vi "set_in_library.vi"(2 "Cluster":T4, 3 "camera cluster":T3, 4 "Tracker Handle":i32, 5 "Array":dbl[][](array[numeric])) -> (0 "No Error":bool, 1 "Directory Exists?":bool)   [LabVIEW 2015]
uses:
  <vilib>/vision/Avi1.llb/AviRefnum.ctl
  <vilib>/userdefined/High Color/IMAQdx.ctl
  MWT.dll
panel:
  out "return type 9":i32
  out "return type 8":i32
  out "return type 7":i32
  out "return type 6":i32
  out "return type 5":i32
  out "return type 4":i32
  out "return type 3":i32
  out "return type 2":i32
  out "return type":i32
  in  "ObjectFrames of Persistence":i32=5
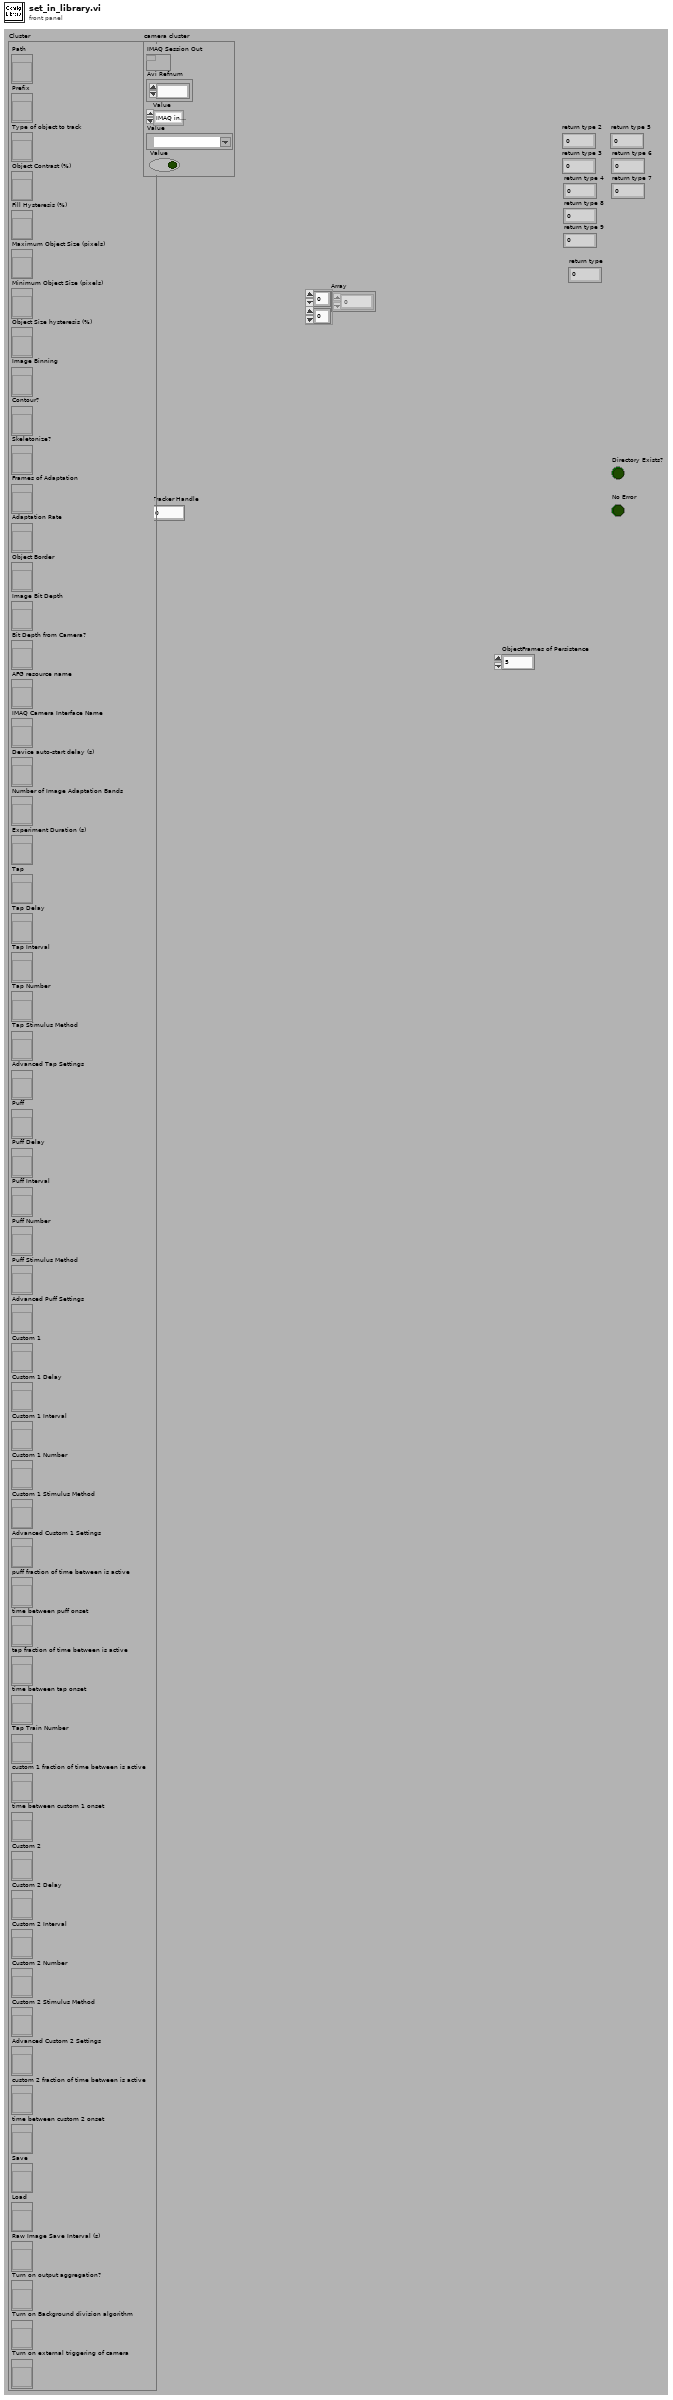
[diagram p1: front panel]
types:
  T1 = typedef "AviRefnum.ctl" = refnum<k1>
  T2 = typedef "IMAQdx.ctl" = refnum<k21>
  T3 = cluster{"IMAQ Session Out":refnum<k11>, "Avi Refnum":T1, "Value":enum32{"IMAQ interface", "IMAQdx interface", "AVI file"}, "Value":T2, "Value":bool}
  T4 = cluster{"Path":refnum<vi>, "Prefix":refnum<vi>, "Type of object to track":refnum<vi>, "Object Contrast (%)":refnum<vi>, "Fill Hysteresis (%)":refnum<vi>, "Maximum Object Size (pixels)":refnum<vi>, "Minimum Object Size (pixels)":refnum<vi>, "Object Size hysteresis (%)":refnum<vi>, "Image Binning":refnum<vi>, "Contour?":refnum<vi>, "Skeletonize?":refnum<vi>, "Frames of Adaptation":refnum<vi>, "Adaptation Rate":refnum<vi>, "Object Border":refnum<vi>, "Image Bit Depth":refnum<vi>, "Bit Depth from Camera?":refnum<vi>, "AFG resource name":refnum<vi>, "IMAQ Camera Interface Name":refnum<vi>, "Device auto-start delay (s)":refnum<vi>, "Number of Image Adaptation Bands":refnum<vi>, "Experiment Duration (s)":refnum<vi>, "Tap":refnum<vi>, "Tap Delay":refnum<vi>, "Tap Interval":refnum<vi>, "Tap Number":refnum<vi>, "Tap Stimulus Method":refnum<vi>, "Advanced Tap Settings":refnum<vi>, "Puff":refnum<vi>, "Puff Delay":refnum<vi>, "Puff Interval":refnum<vi>, "Puff Number":refnum<vi>, "Puff Stimulus Method":refnum<vi>, "Advanced Puff Settings":refnum<vi>, "Custom 1":refnum<vi>, "Custom 1 Delay":refnum<vi>, "Custom 1 Interval":refnum<vi>, "Custom 1 Number":refnum<vi>, "Custom 1 Stimulus Method":refnum<vi>, "Advanced Custom 1 Settings":refnum<vi>, "puff fraction of time between is active":refnum<vi>, "time between puff onset":refnum<vi>, "tap fraction of time between is active":refnum<vi>, "time between tap onset":refnum<vi>, "Tap Train Number":refnum<vi>, "custom 1 fraction of time between is active":refnum<vi>, "time between custom 1 onset":refnum<vi>, "Custom 2":refnum<vi>, "Custom 2 Delay":refnum<vi>, "Custom 2 Interval":refnum<vi>, "Custom 2 Number":refnum<vi>, "Custom 2 Stimulus Method":refnum<vi>, "Advanced Custom 2 Settings":refnum<vi>, "custom 2 fraction of time between is active":refnum<vi>, "time between custom 2 onset":refnum<vi>, "Save":refnum<vi>, "Load":refnum<vi>, "Raw Image Save Interval (s)":refnum<vi>, "Turn on output aggregation?":refnum<vi>, "Turn on Background division algorithm":refnum<vi>, "Turn on external triggering of camera":refnum<vi>}
  T5 = cluster{"Value":path, "Value":string, "Value":bool, "Value":dbl, "Value":dbl, "Value":i32, "Value":i32, "Value":dbl, "Value":u16, "Value":bool, "Value":bool, "Value":i32, "Value":i32, "Value":i32, "Value":u32, "Value":i32, "Value":bool}
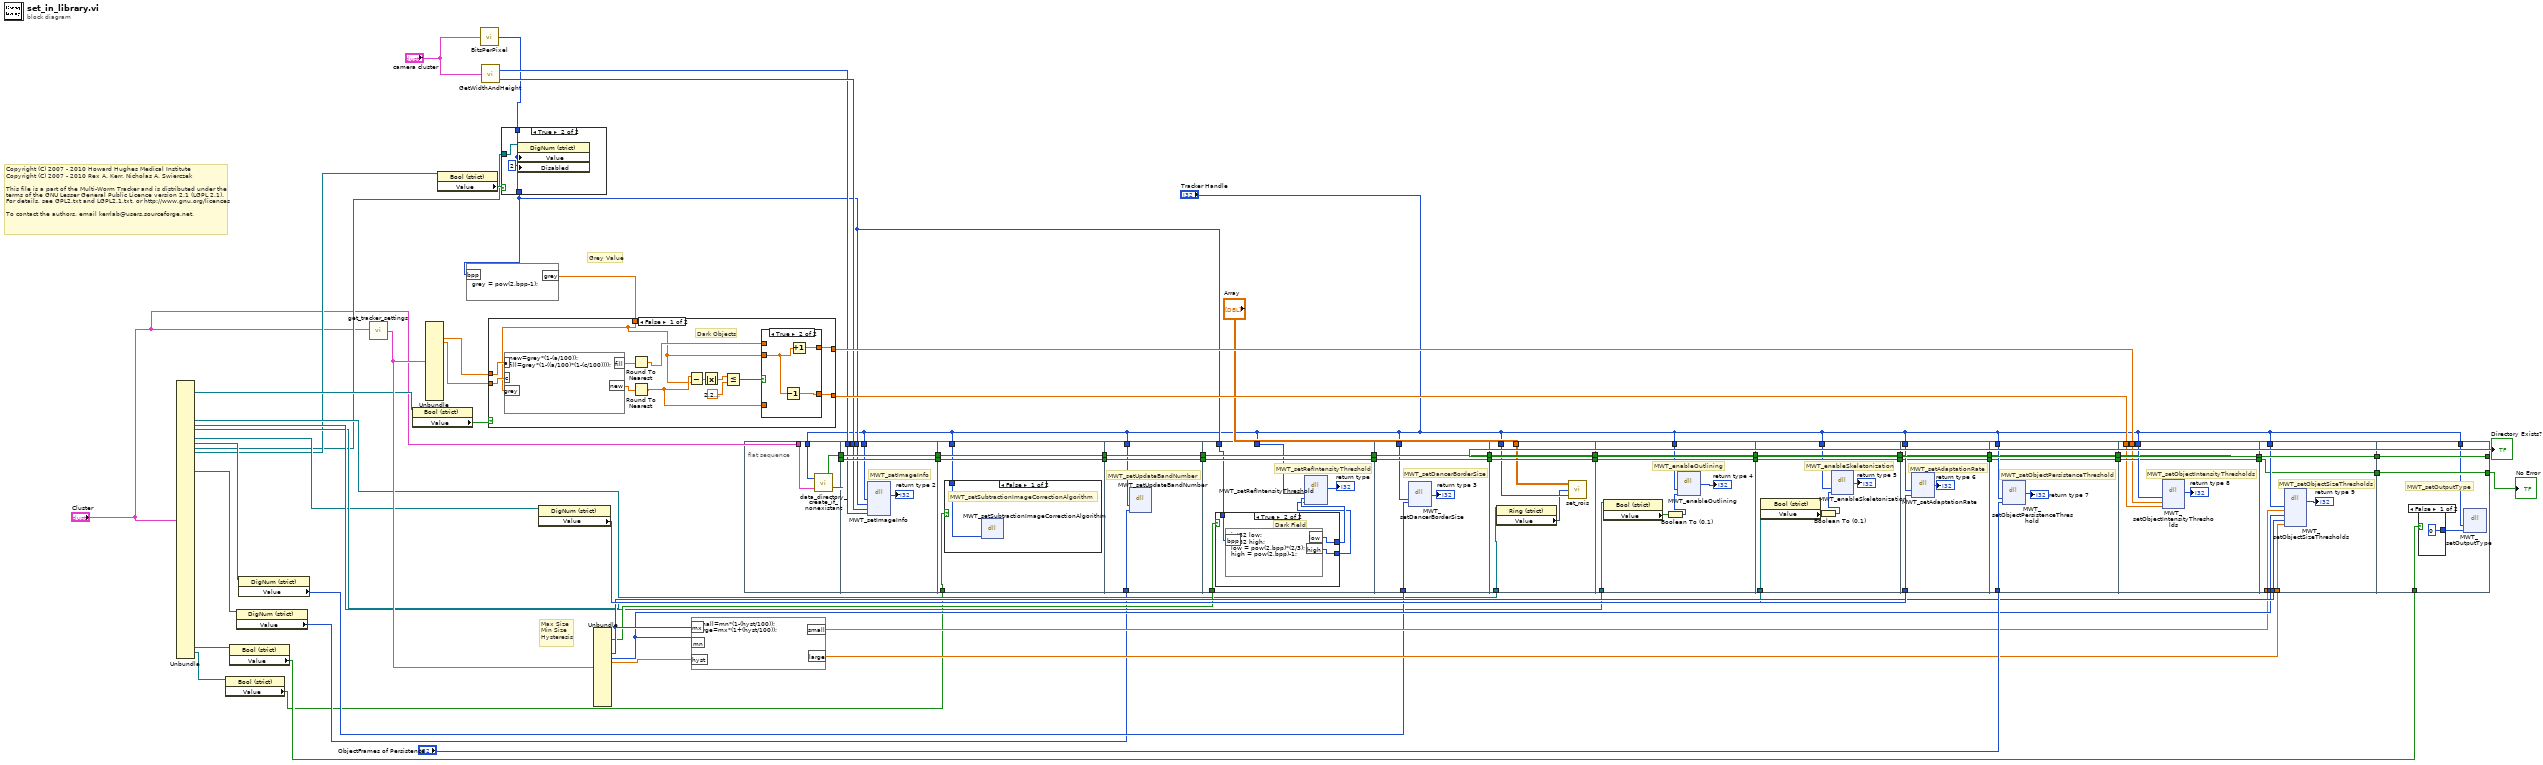
[diagram p0: block diagram]
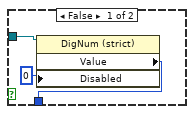
[diagram p2: hidden frame]
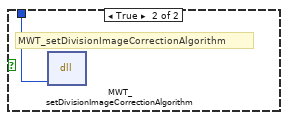
[diagram p3: hidden frame]
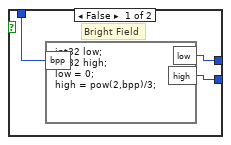
[diagram p4: hidden frame]
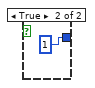
[diagram p5: hidden frame]
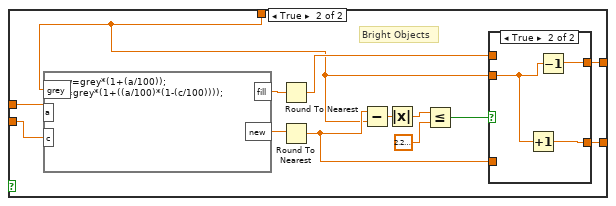
[diagram p7: hidden frame]
diagram:
  # "Copyright (C) 2007 - 2010 Howard Hughes Medical Institute\nCopyright (C) 2007 - 2010 Rex A. Kerr, Nicholas A. Swierczek\n \nThis file is a part of the Multi-Worm Tracker and is distributed under the\nterms of the GNU Lesser General Public Licence version 2.1 (LGPL 2.1).\nFor details, see GPL2.txt and LGPL2.1.txt, or http://www.gnu.org/licences\n \nTo contact the authors, email kerrlab@users.sourceforge.net."
  # "Max Size\nMin Size\nHysteresis"
  # "Grey Value"
  n1 = Unbundle("Cluster") -> ("Type of object to track"=w25:refnum<vi>, "Image Binning"=w24:refnum<vi>, "Contour?"=w23:refnum<vi>, "Skeletonize?"=w22:refnum<vi>, "Adaptation Rate"=w21:refnum<vi>, "Object Border"=w20:refnum<vi>, "Image Bit Depth"=w18:refnum<vi>, "Bit Depth from Camera?"=w19:refnum<vi>, "Number of Image Adaptation Bands"=w15:refnum<vi>, "Turn on output aggregation?"=w11:refnum<vi>, "Turn on Background division algorithm"=w5:refnum<vi>)  [unwired: 49 out]
  n2 = property class="Bool (strict)"(reference=w5) -> ("Value"=w4:bool)  [unwired: 1 in, 2 out]
  n3 = property class="Bool (strict)"(reference=w11) -> ("Value"=w10:bool)  [unwired: 1 in, 2 out]
  n4 = property class="DigNum (strict)"(reference=w15) -> ("Value"=w14:i32)  [unwired: 1 in, 2 out]
  n5 = property class="DigNum (strict)"(reference=w20) -> ("Value"=w31:i32)  [unwired: 1 in, 2 out]
  n6 = call "get_tracker_settings.vi"("Cluster"="Cluster") -> ("settings value cluster"=w66:T5)
  n7 = property class="Bool (strict)"(reference=w25) -> ("Value"=w67:bool)  [unwired: 1 in, 2 out]
  n8 = Unbundle(w66) -> ("Value"=w37:dbl, "Value"=w65:dbl)  [unwired: 15 out]
  n9 = property class="Bool (strict)"(reference=w19) -> ("Value"=w42:bool)  [unwired: 1 in, 2 out]
  n10 = call "BitsPerPixel.vi"("camera cluster"="camera cluster") -> ("BitsPerPixel"=w28:u32)
  n11 = call "GetWidthAndHeight.vi"("camera cluster"="camera cluster") -> ("Width"=w29:u32, "Height"=w30:u32)
  n12 = case shown="True" w42 {
    tunnel: [w69 w72] -> w27
    tunnel: w28 -> [_ w72]
    tunnel: w18 -> [w70 w73]
    frame False {
      n13 = property class="DigNum (strict)"(reference=w70, "Disabled"=u8 0) -> ("Value"=w69:u32)  [unwired: 1 in, 2 out]
    }
    frame True {
      n14 = property class="DigNum (strict)"(reference=w73, "Value"=w72, "Disabled"=u8 2) -> ()  [unwired: 1 in, 2 out]
    }
  }
  n15 = formula code="grey = pow(2,bpp-1);"("bpp"=w27) -> ("grey"=w43:dbl)
  n16 = case shown="False" w67 {
    tunnel: w43 -> [w74 w92]
    tunnel: w37 -> [w86 w104]
    tunnel: w65 -> [w85 w103]
    tunnel: [w77 w100] -> w64
    tunnel: [w78 w98] -> w63
    frame False {
      # "Dark Objects"
      n17 = formula code="new=grey*(1-(a/100));\nfill=grey*(1-((a/100)*(1-(c/100))));"("a"=w86, "c"=w85, "grey"=w74) -> ("new"=w84:dbl, "fill"=w83:dbl)
      n18 = Round To Nearest(number=w83) -> (nearest integer value=w76:dbl)
      n19 = Round To Nearest(number=w84) -> (nearest integer value=w75:dbl)
      n20 = Subtract(x=w75, y=w74) -> (x-y=w82:dbl)
      n21 = Absolute Value(x=w82) -> (abs(x)=w80:dbl)
      n22 = Less Or Equal?(x=w80, y=2.220446049250313e-16) -> (x <= y?=w81:bool)
      n23 = case shown="True" w81 {
        tunnel: [w88 w90] -> w77
        tunnel: w76 -> [w88 _]
        tunnel: [w87 w91] -> w78
        tunnel: w75 -> [w87 _]
        tunnel: w74 -> [_ w89]
        frame False {
        }
        frame True {
          n24 = Decrement(x=w89) -> (x-1=w91:dbl)
          n25 = Increment(x=w89) -> (x+1=w90:dbl)
        }
      }
    }
    frame True {
      # "Bright Objects"
      n26 = formula code="new=grey*(1+(a/100));\nfill=grey*(1+((a/100)*(1-(c/100))));"("a"=w104, "c"=w103, "grey"=w92) -> ("new"=w102:dbl, "fill"=w101:dbl)
      n27 = Round To Nearest(number=w101) -> (nearest integer value=w99:dbl)
      n28 = Round To Nearest(number=w102) -> (nearest integer value=w96:dbl)
      n29 = Subtract(x=w96, y=w92) -> (x-y=w97:dbl)
      n30 = Absolute Value(x=w97) -> (abs(x)=w94:dbl)
      n31 = Less Or Equal?(x=w94, y=2.220446049250313e-16) -> (x <= y?=w95:bool)
      n32 = case shown="True" w95 {
        tunnel: [w106 w108] -> w100
        tunnel: w99 -> [w106 _]
        tunnel: [w105 w109] -> w98
        tunnel: w96 -> [w105 _]
        tunnel: w92 -> [_ w107]
        frame False {
        }
        frame True {
          n33 = Increment(x=w107) -> (x+1=w109:dbl)
          n34 = Decrement(x=w107) -> (x-1=w108:dbl)
        }
      }
    }
  }
  n35 = property class="DigNum (strict)"(reference=w21) -> ("Value"=w62:i32)  [unwired: 1 in, 2 out]
  n36 = Unbundle(w66) -> ("Value"=w26:bool, "Value"=w36:i32, "Value"=w35:i32, "Value"=w34:dbl)  [unwired: 13 out]
  n37 = formula code="small=mn*(1-(hyst/100));\nlarge=mx*(1+(hyst/100));"("mx"=w36, "mn"=w35, "hyst"=w34) -> ("small"=w33:dbl, "large"=w32:dbl)
  n38 = flat-sequence {
    tunnel: [w113] -> w45
    tunnel: [w112] -> w44
    tunnel: "Tracker Handle" -> [w111]
    tunnel: "Cluster" -> [w110]
    tunnel: w45 -> [w120]
    tunnel: [w120] -> w9
    tunnel: w44 -> [w119]
    tunnel: [w119] -> w7
    tunnel: "Tracker Handle" -> [w118]
    tunnel: w27 -> [w117]
    tunnel: w29 -> [w116]
    tunnel: w30 -> [w115]
    tunnel: w9 -> [w124]
    tunnel: [w124] -> w8
    tunnel: w7 -> [w123]
    tunnel: [w123] -> w6
    tunnel: w4 -> [w122]
    tunnel: "Tracker Handle" -> [w121]
    tunnel: w8 -> [w130]
    tunnel: [w130] -> w17
    tunnel: w6 -> [w129]
    tunnel: [w129] -> w16
    tunnel: "Tracker Handle" -> [w128]
    tunnel: w14 -> [w127]
    tunnel: w17 -> [w138]
    tunnel: [w138] -> w49
    tunnel: w16 -> [w137]
    tunnel: [w137] -> w47
    tunnel: "Tracker Handle" -> [w136]
    tunnel: w27 -> [w133]
    tunnel: w26 -> [w134]
    tunnel: w49 -> [w149]
    tunnel: [w149] -> w48
    tunnel: w47 -> [w148]
    tunnel: [w148] -> w46
    tunnel: "Tracker Handle" -> [w147]
    tunnel: w31 -> [w146]
    tunnel: w48 -> [w155]
    tunnel: [w155] -> w41
    tunnel: w46 -> [w154]
    tunnel: [w154] -> w39
    tunnel: "Array" -> [w153]
    tunnel: "Tracker Handle" -> [w152]
    tunnel: w24 -> [w151]
    tunnel: w41 -> [w162]
    tunnel: [w162] -> w40
    tunnel: w39 -> [w161]
    tunnel: [w161] -> w38
    tunnel: "Tracker Handle" -> [w158]
    tunnel: w23 -> [w157]
    tunnel: [w169] -> w57
    tunnel: w40 -> [w169]
    tunnel: w38 -> [w168]
    tunnel: [w168] -> w56
    tunnel: "Tracker Handle" -> [w167]
    tunnel: w22 -> [w166]
    tunnel: w62 -> [w174]
    tunnel: "Tracker Handle" -> [w173]
    tunnel: [w172] -> w58
    tunnel: w57 -> [w172]
    tunnel: w56 -> [w171]
    tunnel: [w171] -> w55
    tunnel: "ObjectFrames of Persistence" -> [w179]
    tunnel: "Tracker Handle" -> [w178]
    tunnel: [w177] -> w59
    tunnel: w58 -> [w177]
    tunnel: w55 -> [w176]
    tunnel: [w176] -> w54
    tunnel: w64 -> [w181]
    tunnel: w63 -> [w182]
    tunnel: "Tracker Handle" -> [w185]
    tunnel: [w184] -> w60
    tunnel: w59 -> [w184]
    tunnel: w54 -> [w183]
    tunnel: [w183] -> w53
    tunnel: w33 -> [w193]
    tunnel: w35 -> [w192]
    tunnel: w36 -> [w191]
    tunnel: w32 -> [w190]
    tunnel: "Tracker Handle" -> [w189]
    tunnel: w60 -> [w188]
    tunnel: w53 -> [w187]
    tunnel: [w188] -> w13
    tunnel: [w187] -> w12
    tunnel: [w197] -> w51
    tunnel: [w198] -> w52
    tunnel: w13 -> [w198]
    tunnel: w12 -> [w197]
    tunnel: "Tracker Handle" -> [w195]
    tunnel: w10 -> [w194]
    frame #0 {
      n39 = call "data_directory_create_if_nonexistant.vi"("Cluster"=w110, "Tracker Handle"=w111) -> ("Error"=w112:bool, "Directory Exists?"=w113:bool)
    }
    frame #1 {
      # "MWT_setImageInfo"
      n40 = dll-call lib="C:/Users/ramasamyl/Desktop/MWT/MWT.dll" fn="MWT_setImageInfo"("handle"=w118, "bits"=w117, "width"=w115, "height"=w116) -> ("return type"=→"return type 2":i32)  [unwired: 7 in, 2 out]
    }
    frame #2 {
      n41 = case shown="False" w122 {
        tunnel: w121 -> [w125 w126]
        frame False {
          # "MWT_setSubtractionImageCorrectionAlgorithm"
          n42 = dll-call lib="C:/Users/ramasamyl/Desktop/MWT/MWT.dll" fn="MWT_setSubtractionImageCorrectionAlgorithm"("handle"=w125) -> ()  [unwired: 5 in, 2 out]
        }
        frame True {
          # "MWT_setDivisionImageCorrectionAlgorithm"
          n43 = dll-call lib="C:/Users/ramasamyl/Desktop/MWT/MWT.dll" fn="MWT_setDivisionImageCorrectionAlgorithm"("handle"=w126) -> ()  [unwired: 5 in, 2 out]
        }
      }
    }
    frame #3 {
      # "MWT_setUpdateBandNumber"
      n44 = dll-call lib="C:/Users/ramasamyl/Desktop/MWT/MWT.dll" fn="MWT_setUpdateBandNumber"("handle"=w128, "num_bands"=w127) -> ()  [unwired: 6 in, 2 out]
    }
    frame #4 {
      # "MWT_setRefIntensityThreshold"
      n45 = case shown="True" w134 {
        tunnel: [w141 w144] -> w132
        tunnel: [w140 w143] -> w131
        tunnel: w133 -> [w139 w142]
        frame False {
          # "Bright Field"
          n46 = formula code="int32 low;\nint32 high;\nlow = 0;\nhigh = pow(2,bpp)/3;"("bpp"=w139) -> ("low"=w141:i32, "high"=w140:i32)
        }
        frame True {
          # "Dark Field"
          n47 = formula code="int32 low;\nint32 high;\nlow = pow(2,bpp)*(2/3);\nhigh = pow(2,bpp)-1;"("bpp"=w142) -> ("low"=w144:i32, "high"=w143:i32)
        }
      }
      n48 = dll-call lib="C:/Users/ramasamyl/Desktop/MWT/MWT.dll" fn="MWT_setRefIntensityThreshold"("handle"=w136, "intensity_low"=w132, "intensity_high"=w131) -> ("return type"=→"return type":i32)  [unwired: 6 in, 2 out]
    }
    frame #5 {
      # "MWT_setDancerBorderSize"
      n49 = dll-call lib="C:/Users/ramasamyl/Desktop/MWT/MWT.dll" fn="MWT_setDancerBorderSize"("handle"=w147, "border_size"=w146) -> ("return type"=→"return type 3":i32)  [unwired: 5 in, 2 out]
    }
    frame #6 {
      n50 = property class="Ring (strict)"(reference=w151) -> ("Value"=w150:u16)  [unwired: 1 in, 2 out]
      n51 = call "set_rois.vi"("Tracker Handle"=w152, "Binning"=w150, "Array"=w153) -> ()
    }
    frame #7 {
      # "MWT_enableOutlining"
      n52 = property class="Bool (strict)"(reference=w157) -> ("Value"=w159:bool)  [unwired: 1 in, 2 out]
      n53 = Boolean To (0,1)(Boolean=w159) -> (0, 1=w160:i16)
      n54 = dll-call lib="C:/Users/ramasamyl/Desktop/MWT/MWT.dll" fn="MWT_enableOutlining"("handle"=w158, "enable"=w160) -> ("return type"=→"return type 4":i32)  [unwired: 5 in, 2 out]
    }
    frame #8 {
      # "MWT_enableSkeletonization"
      n55 = property class="Bool (strict)"(reference=w166) -> ("Value"=w165:bool)  [unwired: 1 in, 2 out]
      n56 = Boolean To (0,1)(Boolean=w165) -> (0, 1=w164:i16)
      n57 = dll-call lib="C:/Users/ramasamyl/Desktop/MWT/MWT.dll" fn="MWT_enableSkeletonization"("handle"=w167, "enable"=w164) -> ("return type"=→"return type 5":i32)  [unwired: 5 in, 2 out]
    }
    frame #9 {
      # "MWT_setAdaptationRate"
      n58 = dll-call lib="C:/Users/ramasamyl/Desktop/MWT/MWT.dll" fn="MWT_setAdaptationRate"("handle"=w173, "alpha"=w174) -> ("return type"=→"return type 6":i32)  [unwired: 5 in, 2 out]
    }
    frame #10 {
      # "MWT_setObjectPersistenceThreshold"
      n59 = dll-call lib="C:/Users/ramasamyl/Desktop/MWT/MWT.dll" fn="MWT_setObjectPersistenceThreshold"("handle"=w178, "frames_of_persistence"=w179) -> ("return type"=→"return type 7":i32)  [unwired: 5 in, 2 out]
    }
    frame #11 {
      # "MWT_setObjectIntensityThresholds"
      n60 = dll-call lib="C:/Users/ramasamyl/Desktop/MWT/MWT.dll" fn="MWT_setObjectIntensityThresholds"("handle"=w185, "intensity_to_fill"=w181, "intensity_of_new"=w182) -> ("return type"=→"return type 8":i32)  [unwired: 6 in, 2 out]
    }
    frame #12 {
      # "MWT_setObjectSizeThresholds"
      n61 = dll-call lib="C:/Users/ramasamyl/Desktop/MWT/MWT.dll" fn="MWT_setObjectSizeThresholds"("handle"=w189, "small_size"=w193, "small_good_size"=w192, "large_good_size"=w191, "large_size"=w190) -> ("return type"=→"return type 9":i32)  [unwired: 8 in, 2 out]
    }
    frame #13 {
      # "MWT_setOutputType"
      n62 = case shown="False" w194 {
        tunnel: [0 1] -> w196
        frame False {
        }
        frame True {
        }
      }
      n63 = dll-call lib="C:/Users/ramasamyl/Desktop/MWT/MWT.dll" fn="MWT_setOutputType"("handle"=w195, "type"=w196) -> ()  [unwired: 6 in, 2 out]
    }
  }
  "Directory Exists?" <- w52
  "No Error" <- w51
